vi "Read Challenge IDs.vi"() -> (0 "error out":errorcluster, 3 "IDs":i32[](array[numeric]))   [LabVIEW 2024, in "Word Search Scorer.lvlib"]
uses:
  Word Search Scorer.lvlib
  <vilib>/Utility/config.llb/NI_LVConfig.lvlib
  <vilib>/Utility/config.llb/Read Key (String).vi
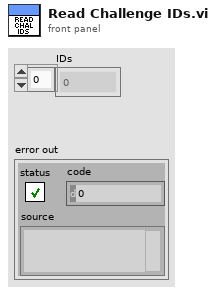
[diagram p1: front panel]
types:
  T1 = typedef "NI_LVConfig.lvlib/Config Data RefNum.ctl" = refnum<k1>
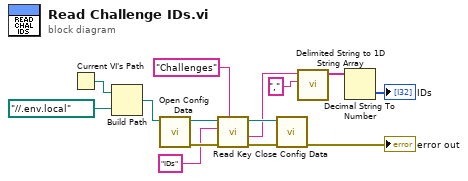
[diagram p0: block diagram]
diagram:
  n1 = Current VI's Path() -> (path=w14:path)
  n2 = Build Path(base path=w14, name or relative path=path "../../.env.local") -> (appended path=w12:path)
  n3 = call <vilib>:"Open Config Data.vi"("configuration file path"=w12) -> ("error out"=w11:errorcluster, "refnum"=w10:T1)  [unwired: 8 in, 1 out]
  n4 = call-poly <vilib>:"Read Key.vi"("section"="Challenges", "error in (no error)"=w11, "key"="IDs", "refnum"=w10) -> ("error out"=w8:errorcluster, "value"=w4:string, "refnum out"=w7:T1)  [unwired: 4 in, 1 out]
  n5 = call <vilib>:"Close Config Data.vi"("error in (no error)"=w8, "refnum"=w7) -> ("error out"=→"error out":errorcluster)  [unwired: 8 in, 1 out]
  n6 = call <vilib>:"Delimited String to 1D String Array.vi"("delimiter"=",", "delimited string"=w4) -> ("string array"=w2:string[])  [unwired: 9 in]
  n7 = Decimal String To Number(string=w2) -> (number=→"IDs":i32[])  [unwired: 2 in, 1 out]
